vi "Display Frequencies LV2016 NI.vi"() -> ()   [LabVIEW 2016]
uses:
  <vilib>/express/express analysis/Spectral/Block/exnSpectralBlock spectral measurements RMS poly.vi
  <vilib>/express/express analysis/Spectral/Block/exnSpectralBlock spectral measurements RMS array WFM.vi
  <vilib>/measure/mamon.llb/Waveform Peak Detection for 1 Chan.vi
  <vilib>/express/express analysis/Spectral/XNode/ExpressSpectralMeasurementsBlockNode.xnode
  <vilib>/measure/NI_MABase.lvlib
  <vilib>/measure/NI_MAPro.lvlib
panel:
  out "FFT Signal":cluster{"f0":dbl, "df":dbl, "magnitude":dbl[]}[](graph)
  out "Frequencies":dbl[][](array[numeric])
  out "Input Signal":waveform(dbl)[](graph)
  # "Overview:\nThis VI shows how to extract the correct frequency values from the output of the Spectral Measurements VI\nRequirements:\nLabVIEW 2012 (or compatible)\nInstructions:\n1. Open DisplayFrequencies.vi\n2. Click Run"
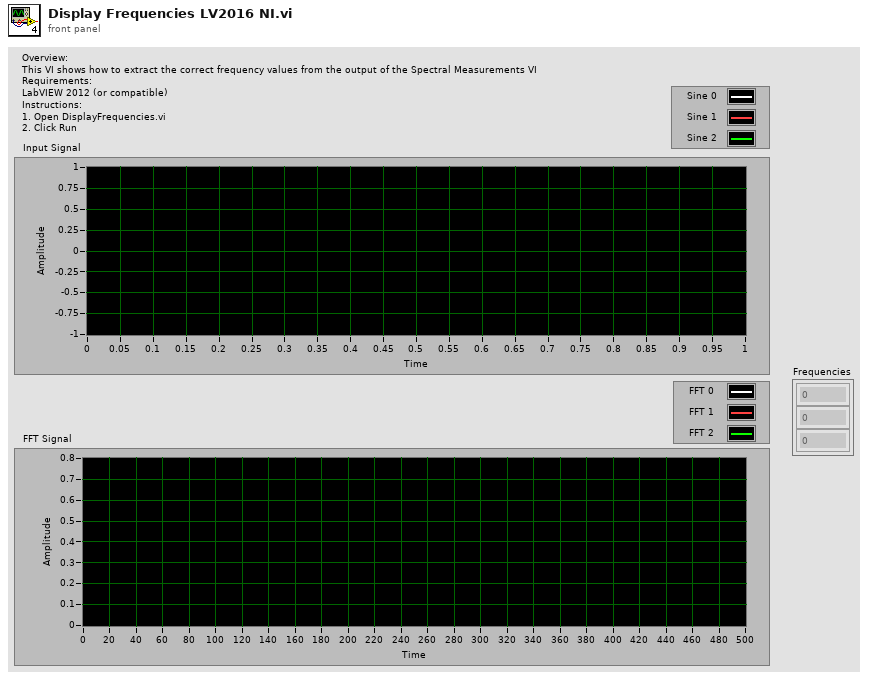
[diagram p1: front panel]
types:
  T1 = enum16{"Sine Wave", "Triangle Wave", "Square Wave", "Sawtooth Wave"}
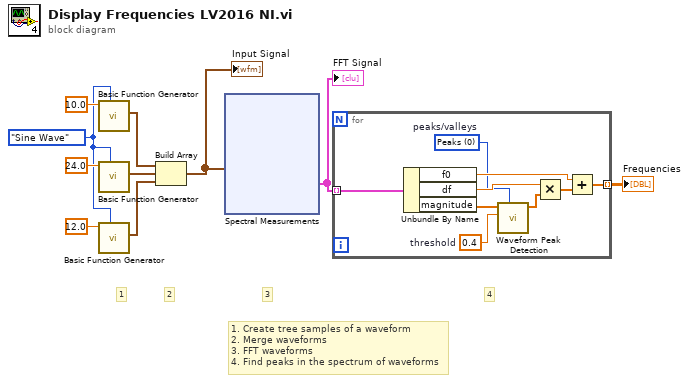
[diagram p0: block diagram]
diagram:
  w7 = T1."Sine Wave" ("signal type")
  # "1. Create tree samples of a waveform\n2. Merge waveforms\n3. FFT waveforms\n4. Find peaks in the spectrum of waveforms"
  # "4"
  # "3"
  # "2"
  # "1"
  n1 = call <vilib>:"Basic Function Generator.vi"("signal type"=w7, "frequency"=10.0) -> ("signal out"=w4:waveform(dbl))  [unwired: 7 in, 2 out]
  n2 = call <vilib>:"Basic Function Generator.vi"("signal type"=w7, "frequency"=24.0) -> ("signal out"=w3:waveform(dbl))  [unwired: 7 in, 2 out]
  n3 = call <vilib>:"Basic Function Generator.vi"("signal type"=w7, "frequency"=12.0) -> ("signal out"=w2:waveform(dbl))  [unwired: 7 in, 2 out]
  n4 = Build Array(w4, w3, w2) -> (w1:waveform(dbl)[])
  "Input Signal" <- w1
  n5 = xnode "Spectral Measurements"("Signals"=w1) -> ("FFT - (RMS)"=w5:cluster{"f0":dbl, "df":dbl, "magnitude":dbl[]}[])  [unwired: 1 in, 2 out]
  "FFT Signal" <- w5
  n6 = for {
    tunnel: w5 -> [w19] mode=indexing
    tunnel: [w11] -> w6 mode=indexing
    w13 = 0.4  # threshold
    w14 = u16 0 items=["Peaks", "Valleys"]  # peaks/valleys
    n7 = Unbundle By Name(w19) -> ("f0"=w16:dbl, "df"=w15:dbl, "magnitude"=w18:dbl[])
    n8 = call-poly <vilib>:"Waveform Peak Detection.vi"("peaks/valleys"=w14, "threshold"=w13, "Signal In"=w18) -> ("Locations"=w12:dbl[])  [unwired: 4 in, 4 out]
    n9 = Multiply(x=w15, y=w12) -> (x*y=w17:dbl[])
    n10 = Add(x=w16, y=w17) -> (x+y=w11:dbl[])
  }
  "Frequencies" <- w6
